vi "New ProjectBuilder.vi"(0 "reference in":refnum<class "ProjectBuilder.lvclass">, 5 "error in (no error)":errorcluster) -> (14 "reference out":refnum<class "ProjectBuilder.lvclass">, 19 "error out":errorcluster)   [LabVIEW 2015, in "ProjectBuilder.lvclass"]
uses:
  ProjectBuilder.lvclass
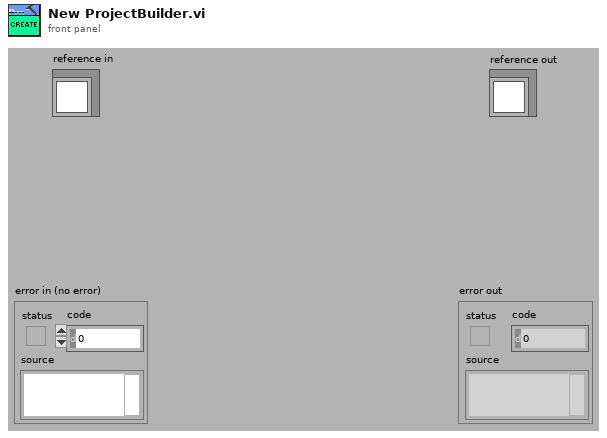
[diagram p1: front panel]
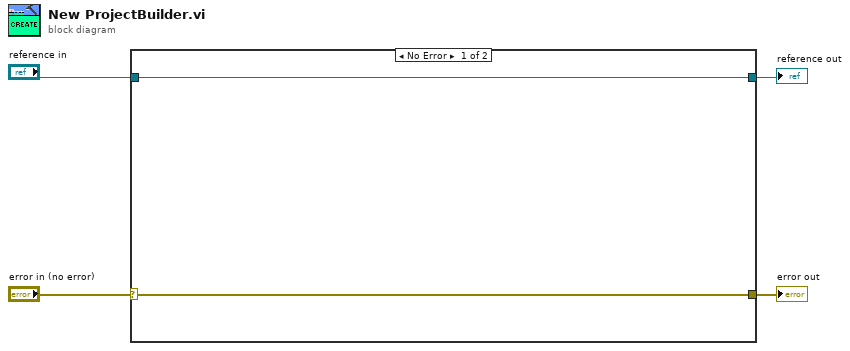
[diagram p0: block diagram]
diagram:
  n1 = case shown="No Error" "error in (no error)" {
    selector: "error in (no error)" -> [w6 w8]
    tunnel: [w6 w8] -> w3
    tunnel: "reference in" -> [w5 w7]
    tunnel: [w5 w7] -> w1
    frame No Error {
    }
    frame Error {
    }
  }
  "error out" <- w3
  "reference out" <- w1
